vi "Parse.vi"(8 "error in (no error)":errorcluster, 11 "PathCommands.CurveTo in":refnum<class "PathCommands.CurveTo.lvclass">) -> (0 "error out":errorcluster, 3 "PathCommands.CurveTo out":refnum<class "PathCommands.CurveTo.lvclass">)   [LabVIEW 2019, in "PathCommands.CurveTo.lvclass"]
uses:
  PathCommands.CurveTo.lvclass
  <vilib>/Utility/error.llb/whitespace.ctl
  PathCommands/Point.ctl
  PathCommands/PathCommands.lvclass
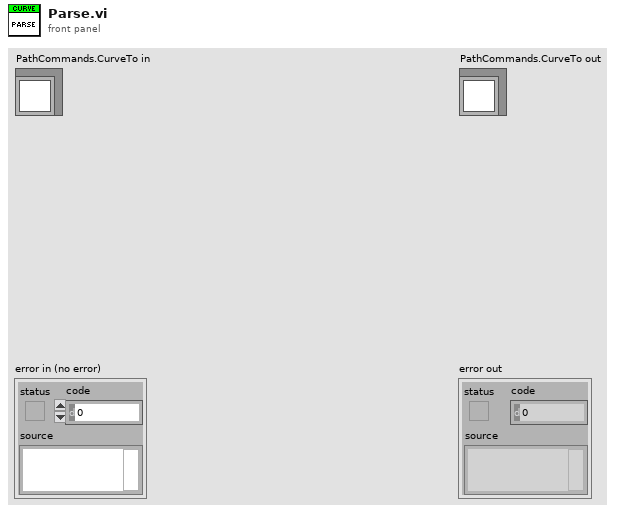
[diagram p1: front panel]
types:
  T1 = typedef "whitespace.ctl" = u16
  T2 = typedef "PathCommands.lvclass/Point.ctl" = cluster{"X":dbl, "Y":dbl}
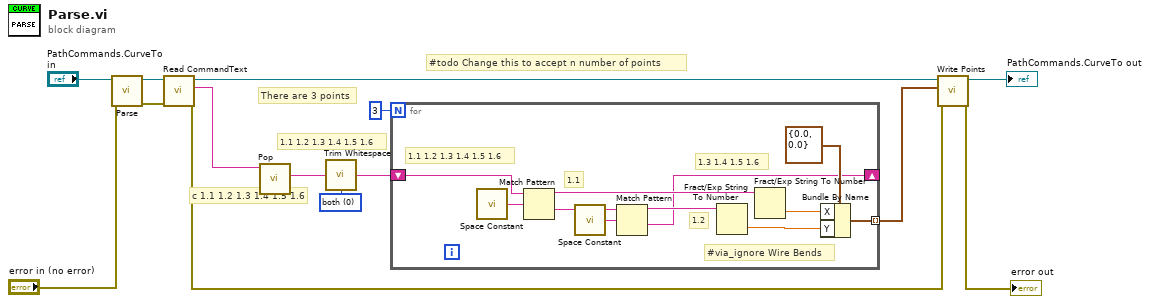
[diagram p0: block diagram]
diagram:
  w9 = T1 0 items=["both", "start of string", "end of string"] ("location (both)")
  # "#todo Change this to accept n number of points"
  # "There are 3 points"
  # "1.1 1.2 1.3 1.4 1.5 1.6"
  # "c 1.1 1.2 1.3 1.4 1.5 1.6"
  n1 = call-parent "Parse.vi"("error in (no error)"="error in (no error)", "PathCommands in"="PathCommands.CurveTo in") -> ("error out"=w5:errorcluster, "PathCommands out"=w12:refnum<class "PathCommands.CurveTo.lvclass">)  [unwired: 8 in]
  n2 = call-dynamic "Read CommandText.vi"("error in (no error)"=w5, "PathCommands in"=w12) -> ("error out"=w4:errorcluster, "CommandText"=w11:string, "PathCommands out"=w8:refnum<class "PathCommands.CurveTo.lvclass">)  [unwired: 7 in]
  n3 = call "Pop.vi"("Command Text"=w11) -> ("Command Info"=w10:string)  [unwired: 9 in, 1 out]
  n4 = call <vilib>:"Trim Whitespace.vi"("string"=w10, "location (both)"=w9) -> ("trimmed string"=w3:string)
  n5 = for {
    N: 3 -> [_]
    tunnel: [w22] -> w1 mode=indexing
    shift-right: [w15] -> _
    shift-left: w3 -> [w16]
    # "#via_ignore Wire Bends"
    # "1.3 1.4 1.5 1.6"
    # "1.1"
    # "1.2"
    # "1.1 1.2 1.3 1.4 1.5 1.6"
    n6 = call <vilib>:"Space Constant.vi"() -> ("String"=w19:string)
    n7 = Match Pattern(string=w16, regular expression=w19) -> (before substring=w17:string, after substring=w20:string)  [unwired: 1 in, 2 out]
    n8 = call <vilib>:"Space Constant.vi"() -> ("String"=w21:string)
    n9 = Match Pattern(string=w20, regular expression=w21) -> (before substring=w18:string, after substring=w15:string)  [unwired: 1 in, 2 out]
    n10 = Fract/Exp String To Number(string=w18) -> (number=w25:dbl)  [unwired: 3 in, 1 out]
    n11 = Fract/Exp String To Number(string=w17) -> (number=w24:dbl)  [unwired: 3 in, 1 out]
    n12 = Bundle By Name(cluster=T2 {"X"=0.0, "Y"=0.0} ("Point"), "X"=w24, "Y"=w25) -> (w22:T2)
  }
  n13 = call-dynamic "Write Points.vi"("error in (no error)"=w4, "Points"=w1, "PathCommands in"=w8) -> ("error out"=→"error out":errorcluster, "PathCommands out"=→"PathCommands.CurveTo out":refnum<class "PathCommands.CurveTo.lvclass">)  [unwired: 7 in]
